vi "Configure Marker_RageATE.vi"(0 "Session In":refnum<visa-resource-name>="TCPIP0::A-N5232A-20122.local::inst0::INSTR", 1 "CH#":i32=1, 5 "MKR#":i32=2, 7 "MKR ON(T)":bool=TRUE, 11 "error in":errorcluster {"code" format="%.0x"}) -> (4 "Session Out":refnum<visa-resource-name>, 10 "error out":errorcluster {"code" format="%.0x"})   [LabVIEW 2018]
doc: "Launches the Instrument I/O Assistant, which you can use to communicate with message-based instruments and graphically parse the response. For example you can communicate with an instrument that uses a serial, Ethernet, or GPIB interface."
panel:
  out "mkr on (t)":bool
  in  "Verify":bool
  # "MAKE SURE THERE IS A MEASUREMENT SELECTED!!!"
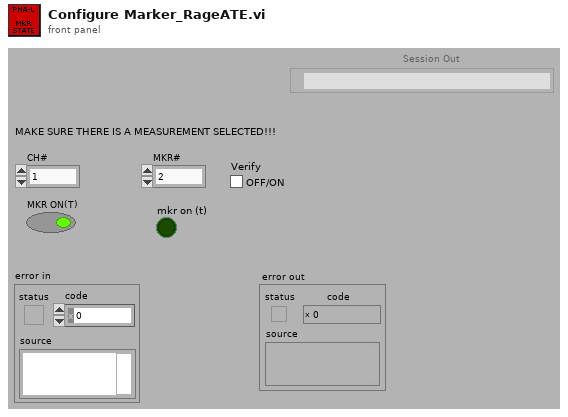
[diagram p1: front panel]
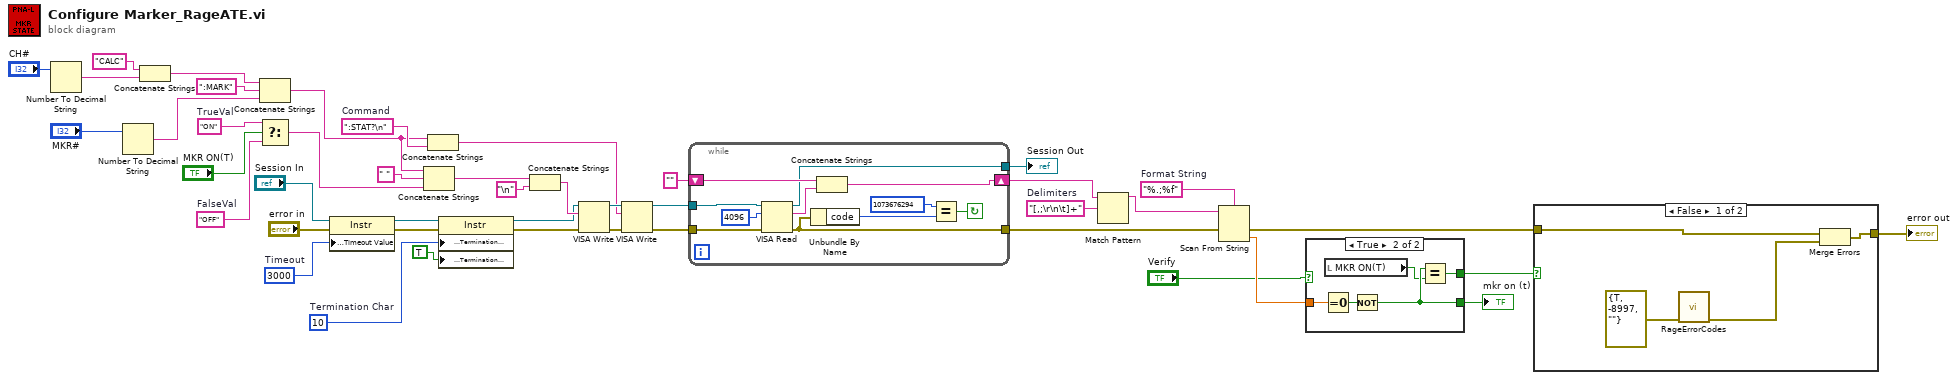
[diagram p0: block diagram]
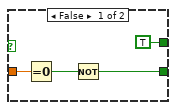
[diagram p3: hidden frame]
diagram:
  w12 = "[,;\r\n\t]+"  # Delimiters
  w13 = "%.;%f"  # Format String
  w16 = ":STAT?\n"  # Command
  w34 = u8 10  # Termination Char
  w38 = u32 3000  # Timeout
  w39 = "OFF"  # FalseVal
  w40 = "ON"  # TrueVal
  n1 = Number To Decimal String(number="CH#") -> (decimal integer string=w31:string)  [unwired: 1 out]
  n2 = Number To Decimal String(number="MKR#") -> (decimal integer string=w29:string)  [unwired: 1 out]
  n3 = Concatenate Strings("CALC" ("staticText"), w31) -> (w28:string)
  n4 = Concatenate Strings(w28, ":MARK" ("staticText"), w29) -> (w7:string)
  n5 = Select(t=w40, s="MKR ON(T)", f=w39) -> (s? t:f=w26:string)
  n6 = property class="Instr"(reference="Session In", error in="error in", "General Settings:Timeout Value"=w38) -> (reference out=w33:refnum<visa-resource-name>, error out=w36:errorcluster)
  n7 = Concatenate Strings(w7, " " ("staticText"), w26) -> (w22:string)
  n8 = Concatenate Strings(w7, w16) -> (w8:string)
  n9 = property class="Instr"(reference=w33, error in=w36, "Message Based Settings:Termination Character"=w34, "Message Based Settings:Termination Character Enable"=TRUE ("enable")) -> (reference out=w11:refnum<visa-resource-name>, error out=w35:errorcluster)
  n10 = Concatenate Strings(w22, "\n" ("StaticText")) -> (w23:string)
  n11 = VISA Write(VISA resource name=w11, write buffer=w23, error in (no error)=w35) -> (VISA resource name out=w10:refnum<visa-resource-name>, error out=w24:errorcluster)  [unwired: 1 out]
  n12 = VISA Write(VISA resource name=w10, write buffer=w8, error in (no error)=w24) -> (VISA resource name out=w20:refnum<visa-resource-name>, error out=w19:errorcluster)  [unwired: 1 out]
  n13 = while {
    tunnel: w20 -> [w52]
    shift-right: [w46] -> w15
    shift-left: "" -> [w51]
    tunnel: w19 -> [w49]
    tunnel: [w48] -> w18
    tunnel: [w45] -> w9
    stop <- w47 continue-if-true
    n14 = VISA Read(VISA resource name=w52, byte count=u32 4096 ("byte count (0)"), error in (no error)=w49) -> (VISA resource name out=w45:refnum<visa-resource-name>, read buffer=w50:string, error out=w48:errorcluster)  [unwired: 1 out]
    n15 = Unbundle By Name(w48) -> ("code"=w54:i32)
    n16 = Concatenate Strings(w51, w50) -> (w46:string)
    n17 = Equal?(x=1073676294, y=w54) -> (x = y?=w47:bool)
  }
  "Session Out" <- w9
  n18 = Match Pattern(string=w15, regular expression=w12) -> (before substring=w14:string)  [unwired: 1 in, 3 out]
  n19 = Scan From String(format string=w13, input string=w14, error in=w18) -> (error out=w2:errorcluster, output 1=w6:dbl)  [unwired: 2 in, 2 out]
  n20 = case shown="True" "Verify" {
    tunnel: w6 -> [w59 w64]
    tunnel: [w57 w62] -> w4
    tunnel: [TRUE w60] -> w1
    frame False {
      n21 = Equal To 0?(x=w59) -> (x = 0?=w58:bool)
      n22 = Not(x=w58) -> (.not. x?=w57:bool)
    }
    frame True {
      n23 = Equal To 0?(x=w64) -> (x = 0?=w63:bool)
      n24 = local read "MKR ON(T)"() -> (w61:bool)
      n25 = Not(x=w63) -> (.not. x?=w62:bool)
      n26 = Equal?(x=w62, y=w61) -> (x = y?=w60:bool)
    }
  }
  "mkr on (t)" <- w4
  n27 = case shown="False" w1 {
    tunnel: [w67 w69] -> w3
    tunnel: w2 -> [w68 w69]
    frame False {
      n28 = call "RageErrorCodes.vi"("error in"=errorcluster {"status"=TRUE, "code"=-8997, "source"=""}) -> ("error out"=w66:errorcluster)  [unwired: 8 in, 2 out]
      n29 = Merge Errors(w68, w66) -> (w67:errorcluster)
    }
    frame True {
    }
  }
  "error out" <- w3
